vi "JSONtext Pretty Print (Colour).vi"(11 "JSON":string) -> (2 "Value String":string, 3 "Boolean":bool)   [LabVIEW 2020]
uses:
  <vilib>/JDP Science/JSONtext/JSONtext.lvlib
panel:
  out "String":string
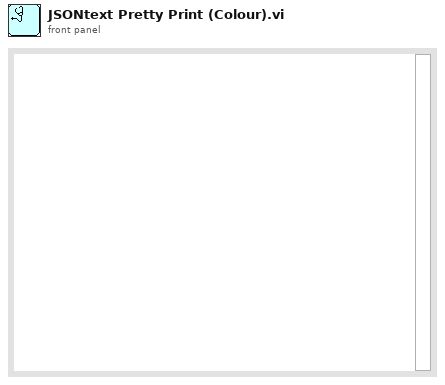
[diagram p1: front panel]
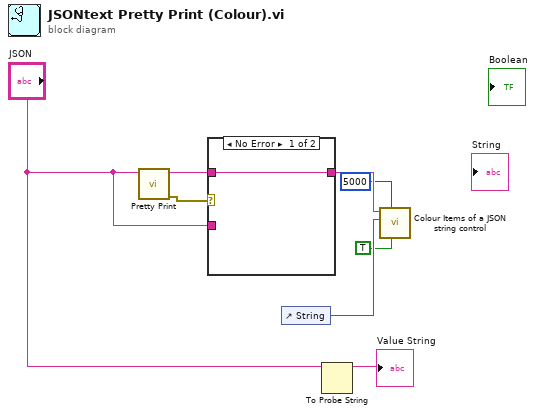
[diagram p0: block diagram]
diagram:
  n1 = call <vilib>:"Pretty Print.vi"("JSON"="JSON") -> ("error out"=w7:errorcluster, "<JSON>"=w6:string)  [unwired: 8 in, 1 out]
  n2 = case shown="No Error" w7 {
    tunnel: [w9 w10] -> w4
    tunnel: w6 -> [w9 _]
    tunnel: "JSON" -> [_ w10]
    frame No Error {
    }
    frame Error {
    }
  }
  n3 = control-ref of="String"() -> (w3:refnum<vi>)
  n4 = To Probe String(7:"JSON") -> (3:→"Value String":string)  [unwired: 2 in, 1 out]
  n5 = call <vilib>:"Colour Items of a JSON string control.vi"("Defer Panel Updates"=TRUE, "Maximum UI Property calls"=5000, "String Control"=w3, "JSON"=w4) -> ()  [unwired: 7 in, 1 out]
